vi "Pane Object Class Tester.vi"() -> ()   [LabVIEW 2018]
uses:
  Pane Object.lvclass/Pane Position Enum.ctl
  Boolean Object.lvclass/Boolean Object Position.lvclass
  Pane Object.lvclass/Pane Object Position.lvclass
panel:
  in  "Magnitude":i32
  out "Direction":enum16{"Right", "Left", "Up", "Down"}(ring)
  out "Nearest Side":T1=enum."Top"
  out "Position":T1=enum."Top"
  in  "Stop":bool
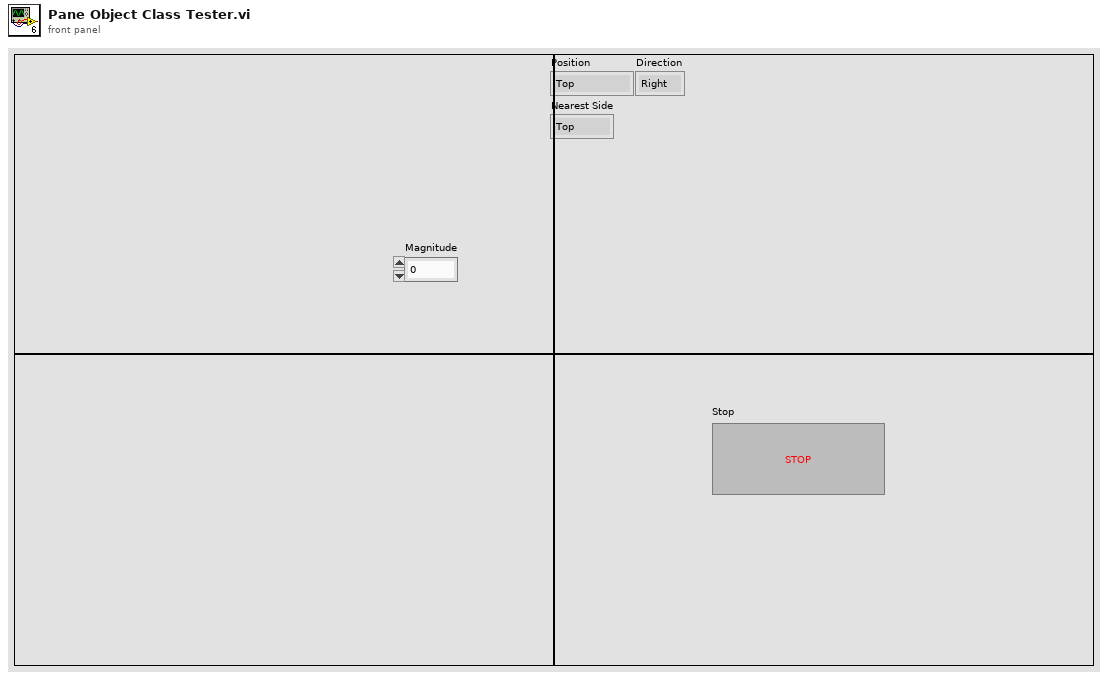
[diagram p1: front panel]
types:
  T1 = typedef "Pane Object Position.lvclass/Pane Position Enum.ctl" = enum16{"Default", "Top", "Right", "Top Right", "Bottom", "5", "Bottom Right", "7", "Left", "Top Left", "10", "11", "Bottom Left"}
  T2 = typedef "Pane Object Position.lvclass/Object Coordinates.ctl" = cluster{"Top":i32, "Right":i32, "Bottom":i32, "Left":i32}
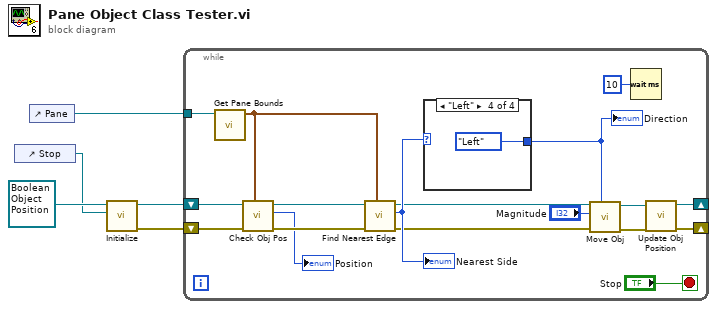
[diagram p0: block diagram]
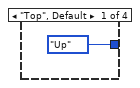
[diagram p2: hidden frame]
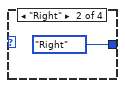
[diagram p3: hidden frame]
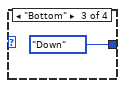
[diagram p4: hidden frame]
diagram:
  n1 = control-ref of="Stop"() -> (w4:refnum<vi>)
  n2 = control-ref of="Pane"() -> (w1:refnum<vi>)
  n3 = call-dynamic "Initialize.vi"("Ctl Refnum"=w4, "Boolean Object Position in"=refnum<class "Boolean Object Position.lvclass"> refnum ("Boolean Object Position.lvclass")) -> ("error out"=w2:errorcluster, "Boolean Object Position out"=w3:refnum<class "Boolean Object Position.lvclass">)  [unwired: 8 in]
  n4 = while {
    tunnel: w1 -> [w21]
    shift-right: [w19] -> _
    shift-left: w3 -> [w23]
    shift-right: [w8] -> _
    shift-left: w2 -> [w22]
    stop <- "Stop" stop-if-true
    n5 = call "Get Pane Bounds.vi"("Pane"=w21) -> ("Panel Coordinates"=w16:T2)  [unwired: 9 in, 1 out]
    n6 = call-dynamic "Check Obj Pos.vi"("Pane Coordinates"=w16, "error in (no error)"=w22, "Boolean Object Position in"=w23) -> ("error out"=w17:errorcluster, "Position"=→"Position":T1, "Boolean Object Position out"=w18:refnum<class "Boolean Object Position.lvclass">)  [unwired: 6 in]
    n7 = call-dynamic "Find Nearest Edge.vi"("Pane Coordinates"=w16, "error in (no error)"=w17, "Boolean Object Position in"=w18) -> ("error out"=w12:errorcluster, "Nearest Side"=w14:T1, "Boolean Object Position out"=w13:refnum<class "Boolean Object Position.lvclass">)  [unwired: 6 in]
    "Nearest Side" <- w14
    n8 = case shown="\"Left\"" w14 {
      tunnel: [enum16{"Right", "Left", "Up", "Down"}."Up" ("Direction") enum16{"Right", "Left", "Up", "Down"}."Right" ("Direction") enum16{"Right", "Left", "Up", "Down"}."Down" ("Direction") enum16{"Right", "Left", "Up", "Down"}."Left" ("Direction")] -> w9
      frame "Top", Default {
      }
      frame "Right" {
      }
      frame "Bottom" {
      }
      frame "Left" {
      }
    }
    "Direction" <- w9
    n9 = call-dynamic "Move Obj.vi"("Direction"=w9, "error in (no error)"=w12, "Magnitude"="Magnitude", "Pane Object Position in"=w13) -> ("error out"=w11:errorcluster, "Pane Object Position out"=w10:refnum<class "Boolean Object Position.lvclass">)  [unwired: 6 in]
    n10 = Wait (ms)(milliseconds to wait=u32 10) -> ()  [unwired: 1 out]
    n11 = call-dynamic "Update Obj Position.vi"("error in (no error)"=w11, "Pane Object Position in"=w10) -> ("error out"=w8:errorcluster, "Pane Object Position out"=w19:refnum<class "Boolean Object Position.lvclass">)  [unwired: 8 in]
  }
